vi "stopReading.vi"(8 "error in (no error)":errorcluster, 10 "Electrometer in":refnum<class "Electrometer.lvclass">, 11 "ReadingState in":refnum<class "ReadingState.lvclass">) -> (0 "error out":errorcluster, 2 "Electrometer out":refnum<class "Electrometer.lvclass">, 3 "ReadingState out":refnum<class "ReadingState.lvclass">)   [LabVIEW 2016, in "ReadingState.lvclass"]
uses:
  ReadingState.lvclass
  Electrometer.lvclass
  GlobalVariables.vi
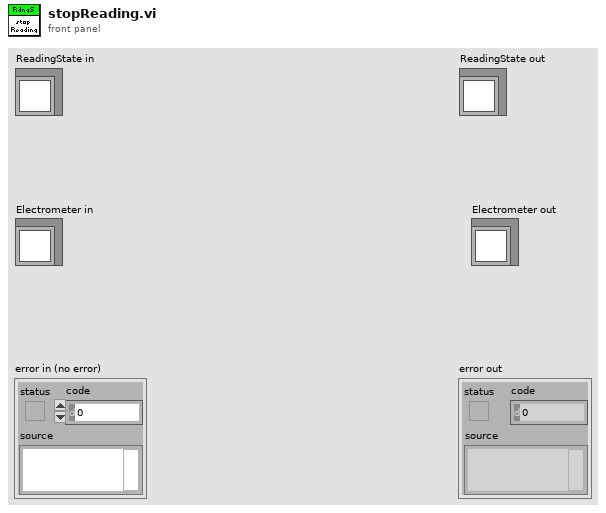
[diagram p1: front panel]
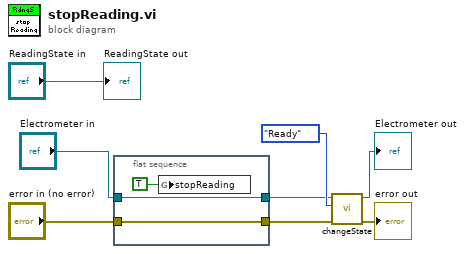
[diagram p0: block diagram]
diagram:
  n1 = flat-sequence {
    tunnel: [w10] -> w4
    tunnel: "error in (no error)" -> [w10]
    tunnel: "Electrometer in" -> [w9]
    tunnel: [w9] -> w2
    frame #0 {
      n2 = global write "GlobalVariables.vi" "stopReading"(TRUE ("stopReading")) -> ()
    }
  }
  n3 = call-dynamic "changeState.vi"("error in (no error)"=w4, "State"=enum16{"Configuring", "Ready", "Reading"}."Ready" ("newState"), "Electrometer in"=w2) -> ("error out"=→"error out":errorcluster, "Electrometer out"=→"Electrometer out":refnum<class "Electrometer.lvclass">)  [unwired: 7 in]
  "ReadingState out" <- "ReadingState in"
